vi "Unflat JSON.vi"(8 "error in (no error)":errorcluster, 10 "JSON string":string, 11 "JSON reader in":refnum<class "JSON reader.lvclass">) -> (0 "error out":errorcluster, 2 "CCD Config":T1, 3 "JSON reader out":refnum<class "JSON reader.lvclass">)   [LabVIEW 2018, in "JSON reader.lvclass"]
uses:
  JSON reader.lvclass
  JSON reader.lvclass/JSON reader.ctl
  Interface/Interface.lvclass
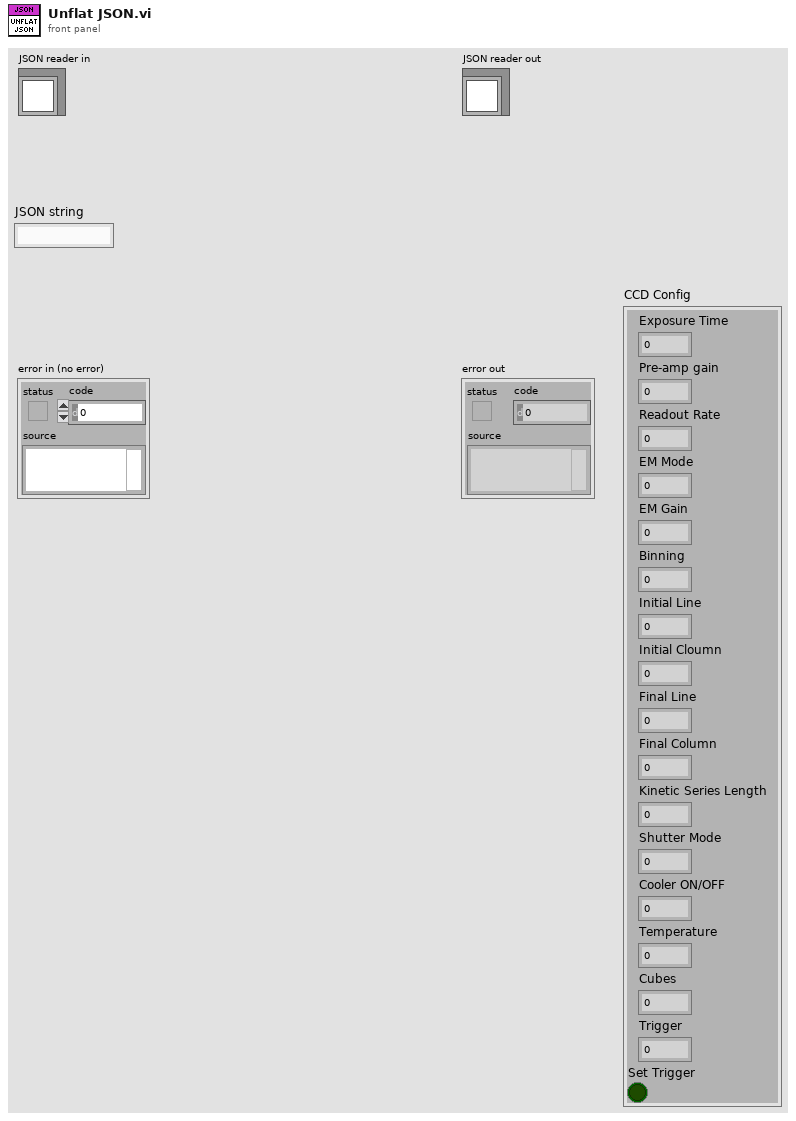
[diagram p1: front panel]
types:
  T1 = cluster{"Exposure Time":sgl, "Pre-amp gain":u8, "Readout Rate":u8, "EM Mode":u8, "EM Gain":u16, "Binning":u16, "Initial Line":u16, "Initial Cloumn":u16, "Final Line":u16, "Final Column":u16, "Kinetic Series Length":u32, "Shutter Mode":u8, "Cooler ON/OFF":u16, "Temperature":i8, "Cubes":u32, "Trigger":u16, "Set Trigger":bool}
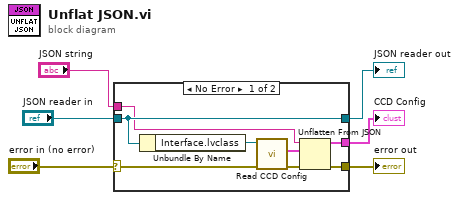
[diagram p0: block diagram]
diagram:
  n1 = case shown="No Error" "error in (no error)" {
    selector: "error in (no error)" -> [w9 w16]
    tunnel: [w12 w16] -> w5
    tunnel: [w14 w15] -> w3
    tunnel: "JSON reader in" -> [w14 w15]
    tunnel: "JSON string" -> [w13 _]
    tunnel: [w11 _] -> w1
    frame No Error {
      n2 = Unbundle By Name(w14) -> ("Interface.lvclass"=w10:refnum<class "Interface.lvclass">)
      n3 = call "Read CCD Config.vi"("error in (no error)"=w9, "Interface in"=w10) -> ("error out"=w8:errorcluster, "CCD Config"=w7:T1)  [unwired: 7 in, 1 out]
      n4 = Unflatten From JSON(JSON string=w13, type and defaults=w7, error in (no error)=w8) -> (value=w11:T1, error out=w12:errorcluster)  [unwired: 4 in]
    }
    frame Error {
    }
  }
  "error out" <- w5
  "JSON reader out" <- w3
  "CCD Config" <- w1
